vi "Adapting_code.vi"(10 "Code":string[](array[string])) -> (2 "Code with an extra dot":string[](array[string]))   [LabVIEW 2022 SP3]
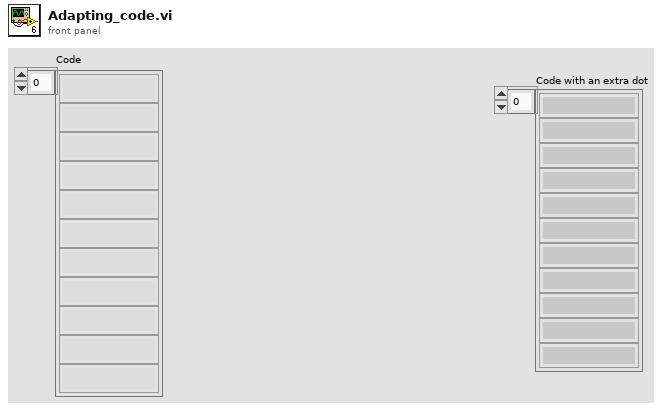
[diagram p1: front panel]
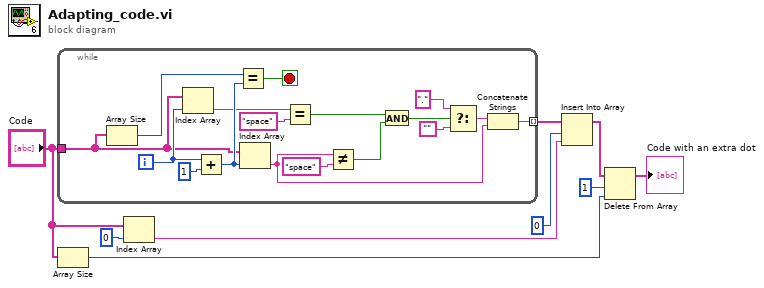
[diagram p0: block diagram]
diagram:
  n1 = while {
    tunnel: "Code" -> [w20]
    tunnel: [w23] -> w9 mode=indexing
    i -> [w21]
    stop <- w24 stop-if-true
    n2 = Array Size(array=w20) -> (size(s)=w25:i32)
    n3 = Index Array(array=w20, index=w21) -> (element=w19:string)
    n4 = Add(x=w21, y=1) -> (x+y=w22:i32)
    n5 = Equal?(x=w25, y=w22) -> (x = y?=w24:bool)
    n6 = Index Array(array=w20, index=w22) -> (element=w11:string)
    n7 = Equal?(x=w19, y="space") -> (x = y?=w13:bool)
    n8 = Not Equal?(x=w11, y="space") -> (x != y?=w10:bool)
    n9 = And(x=w13, y=w10) -> (x .and. y?=w14:bool)
    n10 = Select(t="." ("string"), s=w14, f="") -> (s? t:f=w15:string)
    n11 = Concatenate Strings(w15, w11) -> (w23:string)
  }
  n12 = Array Size(array="Code") -> (size(s)=w1:i32)
  n13 = Index Array(array="Code", index=0) -> (element=w6:string)
  n14 = Insert Into Array(array=w9, index=0, new element=w6) -> (w5:string[])
  n15 = Delete From Array(array=w5, length=1, index=w1) -> (array with subset deleted=→"Code with an extra dot":string[])  [unwired: 1 out]
